vi "Configure Ramp.vi"(0 "VISA resource name":refnum<visa-resource-name>, 5 "Loop (1:Loop 1)":u16(ring)=1 items=["Loop 1"=1, "Loop 2"=2], 7 "Rate Value (0.0)":dbl format="%.1f", 9 "Setpoint Ramp (F: Off)":bool, 11 "error in (no error)":errorcluster) -> (4 "VISA resource name out":refnum<visa-resource-name>, 15 "error out":errorcluster)   [LabVIEW 2019, in "Lake Shore 325.lvlib"]
doc: "This VI configures the setpoint ramp function. The Model 325 generates a smooth setpoint ramp when the setpoint units are expressed in temperature. Once the ramp feature is turned on, its action is initiated by a setpoint change. When a new setpoint is entered, the instrument changes the setpoint temperature from the old value to the new value at the ramp rate."
uses:
  Lake Shore 325.lvlib
  Instance           1 22Saved   Configure Ramp .vi
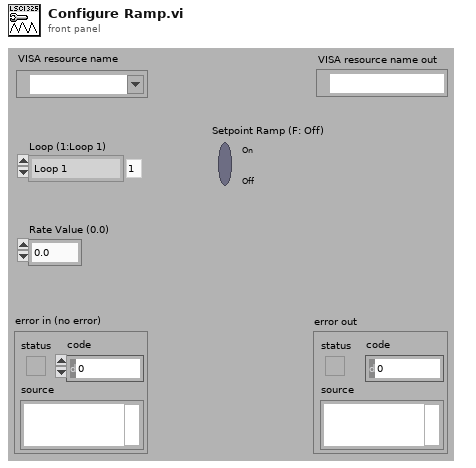
[diagram p1: front panel]
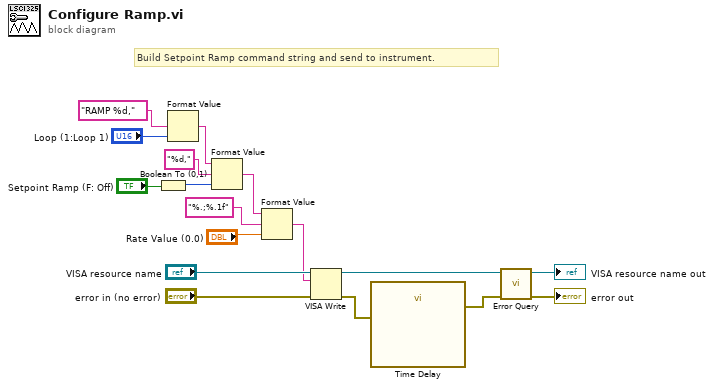
[diagram p0: block diagram]
diagram:
  # "Build Setpoint Ramp command string and send to instrument."
  n1 = Boolean To (0,1)(Boolean="Setpoint Ramp (F: Off)") -> (0, 1=w8:i16)
  n2 = Format Value(format string="RAMP %d,", value (0)="Loop (1:Loop 1)") -> (output string=w9:string)  [unwired: 1 in]
  n3 = Format Value(string ("")=w9, format string="%d,", value (0)=w8) -> (output string=w5:string)
  n4 = Format Value(string ("")=w5, format string="%.;%.1f", value (0)="Rate Value (0.0)") -> (output string=w4:string)
  n5 = VISA Write(VISA resource name="VISA resource name", write buffer=w4, error in (no error)="error in (no error)") -> (VISA resource name out=w15:refnum<visa-resource-name>, error out=w2:errorcluster)  [unwired: 1 out]
  n6 = call "Time Delay"("error in (no error)"=w2) -> ("error out"=w1:errorcluster)  [unwired: 10 in]
  n7 = call "Error Query.vi"("error in (no error)"=w1, "VISA resource name"=w15) -> ("error out"=→"error out":errorcluster, "VISA resource name out"=→"VISA resource name out":refnum<visa-resource-name>)  [unwired: 7 in, 1 out]
